vi "Overlay Match Multiple Geometric Patterns Results.vi"(5 "Overlay Group":string, 6 "Label Colors":u32[](array[colorbox]), 7 "Learned Labels":string[](array[string]), 8 "error in":errorcluster, 9 "Match Labels":string[](array[string]), 10 "Match Results":T1(array[cluster]), 11 "Image":T2) -> (0 "error out":errorcluster, 2 "Number of Matches":i32[](array[numeric]), 3 "Image Out":T2)   [LabVIEW 2017]
uses:
  <vilib>/vision/Image Controls.llb/IMAQ Image.ctl
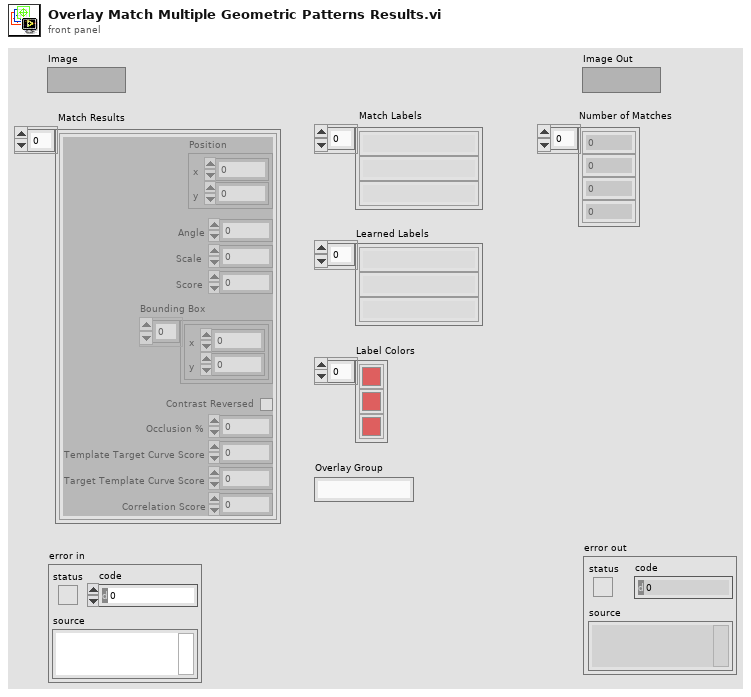
[diagram p1: front panel]
types:
  T1 = cluster{"Position":cluster{"x":sgl, "y":sgl}, "Angle":sgl, "Scale":sgl, "Score":sgl, "Bounding Box":cluster{"x":sgl, "y":sgl}[], "Contrast Reversed":bool, "Occlusion %":sgl, "Template Target Curve Score":sgl, "Target Template Curve Score":sgl, "Correlation Score":sgl}[]
  T2 = typedef "IMAQ Image.ctl" = refnum<image>
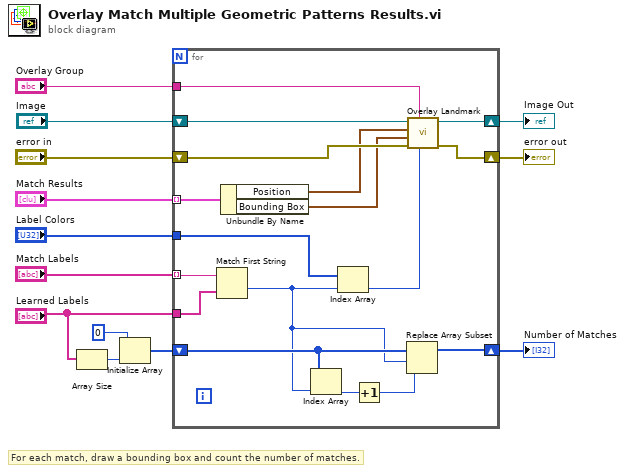
[diagram p0: block diagram]
diagram:
  # "For each match, draw a bounding box and count the number of matches."
  n1 = Array Size(array="Learned Labels") -> (size(s)=w10:i32)
  n2 = Initialize Array(0 ("x+1"), w10) -> (w8:i32[])
  n3 = for {
    shift-right: [w20] -> w13
    shift-left: "Image" -> [w21]
    tunnel: "Match Results" -> [w30] mode=indexing
    tunnel: "Match Labels" -> [w29] mode=indexing
    shift-right: [w27] -> w12
    shift-left: w8 -> [w28]
    tunnel: "Learned Labels" -> [w24]
    shift-right: [w18] -> w3
    shift-left: "error in" -> [w19]
    tunnel: "Label Colors" -> [w17]
    tunnel: "Overlay Group" -> [w14]
    n4 = Match First String(2:w24, 3:w29) -> (0:w23:i32)  [unwired: 1 out]
    n5 = Unbundle By Name(w30) -> ("Position"=w15:cluster{"x":sgl, "y":sgl}, "Bounding Box"=w16:cluster{"x":sgl, "y":sgl}[])
    n6 = Index Array(array=w28, index=w23) -> (element=w26:i32)
    n7 = Index Array(array=w17, index=w23) -> (element=w22:u32)
    n8 = Increment(x=w26) -> (x+1=w25:i32)
    n9 = Replace Array Subset(array=w28, new element=w25, index=w23) -> (w27:i32[])
    n10 = call "Overlay Landmark.vi"("Color"=w22, "Group"=w14, "error in"=w19, "Bounding Box"=w16, "Position"=w15, "Image"=w21) -> ("error out"=w18:errorcluster, "Image Out"=w20:T2)  [unwired: 4 in]
  }
  "Image Out" <- w13
  "Number of Matches" <- w12
  "error out" <- w3
